vi "file_LabVIEW_4b.vi"() -> ()   [LabVIEW 2015]
uses:
  <vilib>/Instr/_visa.llb/VISA Configure Serial Port (Instr).vi
panel:
  in  "SETPOINT":i16(knob) scale=-165.0..165.0
  out "SETPOINT & OUTPUT":cluster{i16, i16}(knob)={0, -52} scale=-165.0..165.0
  out "Grafik Encoder":cluster{"SETPOINT":i16, dbl}(graph)
  out "read buffer":string
  out "Slide":i16(slide) scale=-255.0..255.0
  in  "VISA resource name":refnum<visa-resource-name>
  in  "stop":bool
  out "Grafik PWM":dbl(graph)
  # "KONTROL KECEPATAN"
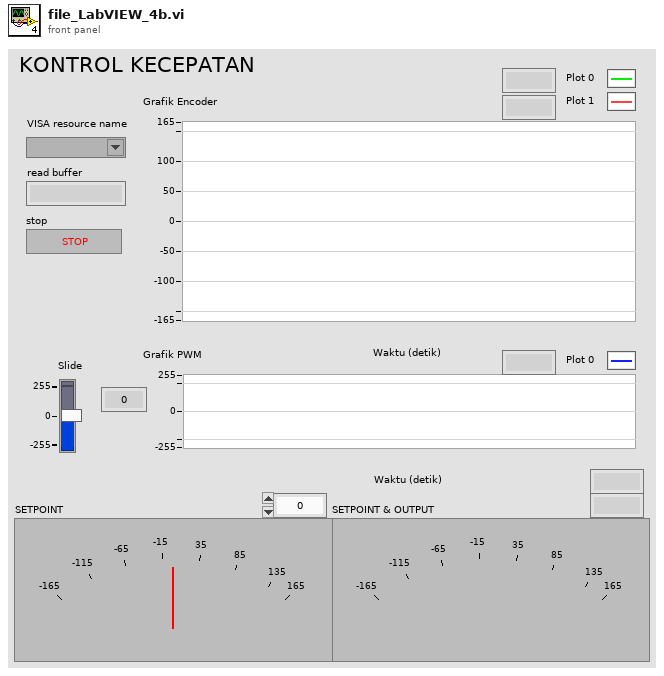
[diagram p1: front panel]
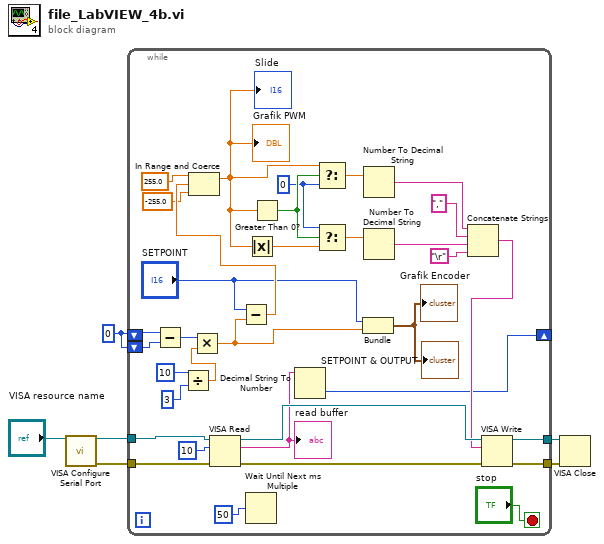
[diagram p0: block diagram]
diagram:
  w1 = 0
  n1 = call-poly "VISA Configure Serial Port"("VISA resource name"="VISA resource name") -> ("VISA resource name out"=w4:refnum<visa-resource-name>, "error out"=w3:errorcluster)  [unwired: 13 in]
  n2 = while {
    tunnel: [w40] -> w6
    tunnel: [w39] -> w5
    tunnel: w4 -> [w27]
    tunnel: w3 -> [w28]
    shift-right: [w14] -> _
    shift-left: w1 -> [w20]
    shift-left: w1 -> [w21]
    stop <- "stop" stop-if-true
    w37 = 0
    n3 = Subtract(x=w20, y=w21) -> (x-y=w19:i32)
    n4 = Divide(x=10, y=3) -> (x/y=w8:dbl)
    n5 = Multiply(x=w19, y=w8) -> (x*y=w13:dbl)
    n6 = VISA Read(VISA resource name=w27, byte count=u32 10, error in (no error)=w28) -> (VISA resource name out=w25:refnum<visa-resource-name>, read buffer=w22:string, error out=w26:errorcluster)  [unwired: 1 out]
    "read buffer" <- w22
    n7 = Subtract(x="SETPOINT", y=w13) -> (x-y=w12:dbl)
    n8 = In Range and Coerce(upper limit=255.0, x=w12, lower limit=-255.0) -> (coerced(x)=w9:dbl)  [unwired: 1 out]
    "Grafik PWM" <- w9
    "Slide" <- w9
    n9 = Wait Until Next ms Multiple(millisecond multiple=u32 50) -> ()  [unwired: 1 out]
    n10 = Absolute Value(x=w9) -> (abs(x)=w36:dbl)
    n11 = Greater Than 0?(x=w9) -> (x > 0?=w38:bool)
    n12 = Decimal String To Number(string=w22) -> (number=w14:i32)  [unwired: 2 in, 1 out]
    n13 = Select(t=w9, s=w38, f=w37) -> (s? t:f=w35:dbl)
    n14 = Select(t=w37, s=w38, f=w36) -> (s? t:f=w34:dbl)
    n15 = Bundle "Bundle"("SETPOINT"="SETPOINT", w13) -> (→"Grafik Encoder" →"SETPOINT & OUTPUT":cluster{"SETPOINT":i16, dbl})  [unwired: 1 in]
    n16 = Number To Decimal String(number=w35) -> (decimal integer string=w33:string)  [unwired: 1 in]
    n17 = Number To Decimal String(number=w34) -> (decimal integer string=w31:string)  [unwired: 1 in]
    n18 = Concatenate Strings "Concatenate Strings"(w33, "," ("string"), w31, "\r") -> (w15:string)
    n19 = VISA Write(VISA resource name=w25, write buffer=w15, error in (no error)=w26) -> (VISA resource name out=w39:refnum<visa-resource-name>, error out=w40:errorcluster)  [unwired: 1 out]
  }
  n20 = VISA Close(VISA resource name=w5, error in (no error)=w6) -> ()  [unwired: 1 out]
